vi "RT message processing.vi"(5 "timeout in ms":i32=5, 6 "error in (no error)":errorcluster, 7 "FPGA VI Reference in":refnum<k20>, 8 "serial message queue":refnum<queue>, 9 "RT message queue":refnum<queue>) -> (0 "error out":errorcluster, 2 "FPGA VI Reference Out":refnum<k20>)   [LabVIEW 2018]
uses:
  Type Def Ctrls/RT ctrls/data summary.ctl
  Message Queue/Message Cluster.ctl
  Type Def Ctrls/RT ctrls/FPGA parameter cluster.ctl
  Type Def Ctrls/FPGA ctrls/NI9219VoltageRange.ctl
  Globals/RT AND FPGA SETTINGS.vi
  Message Queue/Message Queue.lvlib
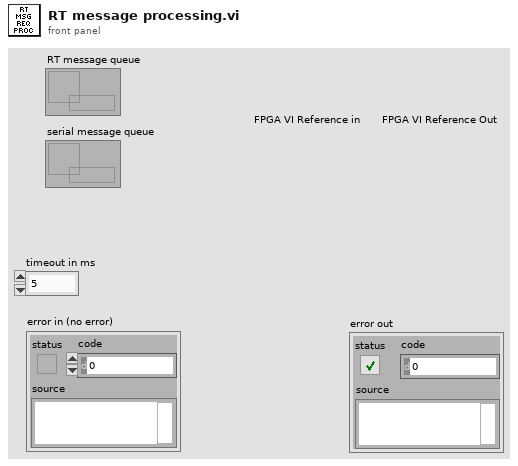
[diagram p1: front panel]
types:
  T1 = typedef "FPGA parameter cluster.ctl" = cluster{"Output settings":cluster{"Relay Switch Matrix":u32, "Set output":sgl[], "set output?":bool, "set relay matrix?":bool}, "PID settings":cluster{"PID input channel":enum16{"Output Channel 0", "Output Channel 1", "Output Channel 2", "Output Channel 3", "PID Disabled"}, "PID output channel":enum16{"Output Channel 0", "Output Channel 1", "Output Channel 2", "Output Channel 3", "PID Disabled"}, "PID gains":cluster{"proportional gain":sgl, "integral gain":sgl, "derivative gain":sgl, "filter coefficient":sgl}, "PID output ranges":cluster{"output high (Inf)":sgl, "output low (-Inf)":sgl}, "Setpoint for PID input chn":sgl, "config PID gain?":bool, "reset PID?":bool, "config PID range?":bool, "config PID input?":bool, "config PID output?":bool, "config PID setpoint?":bool}, "NI9219 Settings":cluster{"9219 Conversion Time":enum8{"High Speed", "Best 60 Hz Rejection", "Best 50 Hz Rejection", "High Resolution"}, "Input voltage range":T2[], "config 9219 conversion time?":bool, "config 9219 input range?":bool}, "REQUEST_ID":u64, "requests":cluster{"request_data":bool, "request_system_status":bool, "request_error_log":bool}}
  T2 = typedef "NI9219VoltageRange.ctl" = u8
  T3 = cluster{"Output settings":cluster{"Relay Switch Matrix":u32, "Set output":sgl[], "set output?":bool, "set relay matrix?":bool}, "PID settings":cluster{"PID input channel":enum16{"Output Channel 0", "Output Channel 1", "Output Channel 2", "Output Channel 3", "PID Disabled"}, "PID output channel":enum16{"Output Channel 0", "Output Channel 1", "Output Channel 2", "Output Channel 3", "PID Disabled"}, "PID gains":cluster{"proportional gain":sgl, "integral gain":sgl, "derivative gain":sgl, "filter coefficient":sgl}, "PID output ranges":cluster{"output high (Inf)":sgl, "output low (-Inf)":sgl}, "Setpoint for PID input chn":sgl, "config PID gain?":bool, "reset PID?":bool, "config PID range?":bool, "config PID input?":bool, "config PID output?":bool, "config PID setpoint?":bool}, "NI9219 Settings":cluster{"9219 Conversion Time":enum8{"High Speed", "Best 60 Hz Rejection", "Best 50 Hz Rejection", "High Resolution"}, "Input voltage range":u8[], "config 9219 conversion time?":bool, "config 9219 input range?":bool}, "REQUEST_ID":u64, "requests":cluster{"request_data":bool, "request_system_status":bool, "request_error_log":bool}}
  T4 = typedef "thermocouple type.ctl" = u16
  T5 = typedef "data summary.ctl" = cluster{"TIMESTAMP":dbl, "INPUT_CHN_DATA":sgl[], "OUTPUT_CHN_DATA":sgl[], "CJC_TEMPERATURE":sgl, "RELAY_SETTING":u32, "REQUEST_ID":u64, "update_system_status?":bool, "update_error_log?":bool}
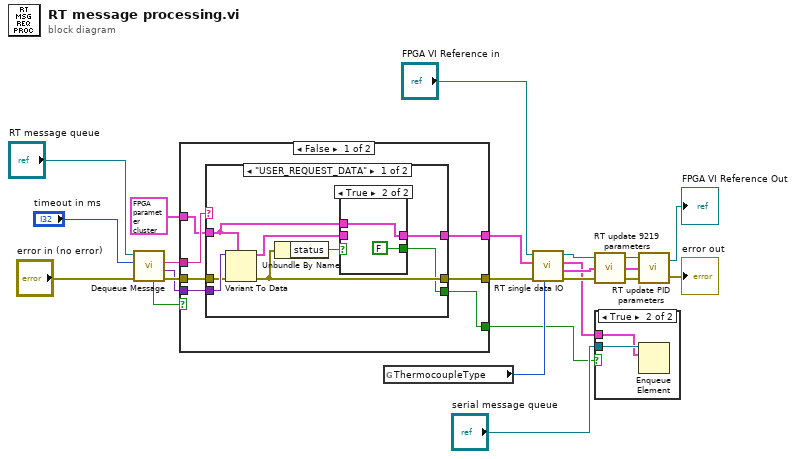
[diagram p0: block diagram]
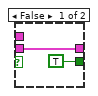
[diagram p3: hidden frame]
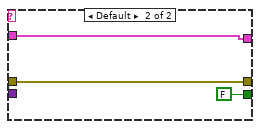
[diagram p4: hidden frame]
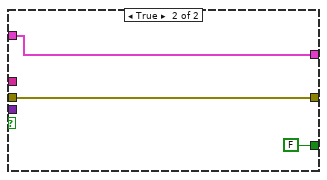
[diagram p5: hidden frame]
diagram:
  n1 = call "Dequeue Message.vi"("error in (no error)"="error in (no error)", "timeout in ms (-1)"="timeout in ms", "Message Queue"="RT message queue") -> ("error out"=w16:errorcluster, "Message Data"=w13:variant, "Message"=w14:string, "timed out?"=w11:bool)  [unwired: 4 in, 1 out]
  n2 = case shown="False" w11 {
    tunnel: w13 -> [w30 _]
    tunnel: w14 -> [w29 _]
    tunnel: [w28 w48] -> w10
    tunnel: T1 {"Output settings"={"Relay Switch Matrix"=0, "Set output"=[0.0, 0.0, 0.0, 0.0], "set output?"=FALSE, "set relay matrix?"=FALSE}, "PID settings"={"PID input channel"=enum."PID Disabled", "PID output channel"=enum."PID Disabled", "PID gains"={"proportional gain"=0.0, "integral gain"=0.0, "derivative gain"=0.0, "filter coefficient"=0.0}, "PID output ranges"={"output high (Inf)"=0.0, "output low (-Inf)"=0.0}, "Setpoint for PID input chn"=0.0, "config PID gain?"=FALSE, "reset PID?"=FALSE, "config PID range?"=FALSE, "config PID input?"=FALSE, "config PID output?"=FALSE, "config PID setpoint?"=FALSE}, "NI9219 Settings"={"9219 Conversion Time"=enum."High Speed", "Input voltage range"=[1, 1, 1, 4], "config 9219 conversion time?"=FALSE, "config 9219 input range?"=FALSE}, "REQUEST_ID"=0, "requests"={"request_data"=FALSE, "request_system_status"=FALSE, "request_error_log"=FALSE}} ("FPGA Parameter cluster") -> [w27 w48]
    tunnel: w16 -> [w26 w47]
    tunnel: [w25 w47] -> w12
    tunnel: [w24 FALSE] -> w2
    frame False {
      n3 = case shown="\"USER_REQUEST_DATA\"" w29 {
        tunnel: w30 -> [w38 _]
        tunnel: [w35 w45] -> w28
        tunnel: w27 -> [w34 w45]
        tunnel: w26 -> [w33 w44]
        tunnel: [w32 w44] -> w25
        tunnel: [w31 FALSE] -> w24
        frame "USER_REQUEST_DATA" {
          n4 = Variant To Data(error in=w33, type=w34, Variant=w38) -> (data=w36:T3, error out=w32:errorcluster)
          n5 = Unbundle By Name(w32) -> ("status"=w37:bool)
          n6 = case shown="True" w37 {
            tunnel: w36 -> [w40 _]
            tunnel: [w40 w42] -> w35
            tunnel: w34 -> [_ w42]
            tunnel: [TRUE FALSE] -> w31
            frame False {
            }
            frame True {
            }
          }
        }
        frame Default {
        }
      }
    }
    frame True {
    }
  }
  n7 = global read "RT AND FPGA SETTINGS.vi" "ThermocoupleType"() -> (w5:T4)
  n8 = call "RT single data IO.vi"("ThermocoupleType"=w5, "error in"=w12, "FPGA Parameter cluster"=w10, "FPGA VI Reference In"="FPGA VI Reference in") -> ("error out"=w9:errorcluster, "FPGA Parameter cluster out"=w4:T1, "data summary"=w1:T5, "FPGA VI Reference Out"=w6:refnum<k20>)  [unwired: 4 in]
  n9 = call "RT update 9219 parameters.vi"("error in"=w9, "FPGA Parameter cluster"=w4, "FPGA VI ref in"=w6) -> ("error out"=w8:errorcluster, "FPGA Parameter cluster out"=w3:T1, "FPGA VI Reference Out"=w7:refnum<k20>)
  n10 = case shown="True" w2 {
    tunnel: "serial message queue" -> [_ w50]
    tunnel: w1 -> [_ w49]
    frame False {
    }
    frame True {
      n11 = Enqueue Element(queue=w50, element=w49) -> ()  [unwired: 2 in, 3 out]
    }
  }
  n12 = call "RT update PID parameters.vi"("error in"=w8, "FPGA Parameter cluster"=w3, "FPGA VI ref in"=w7) -> ("error out"=→"error out":errorcluster, "FPGA VI Reference Out"=→"FPGA VI Reference Out":refnum<k20>)
